vi "ImageManipulationNewLifetimeCalculation.vi"(0 "Array":T1[](array[typedef]) {"F2-Value overall" format="%.2f"; "tauerror" format="%.2f"; "Lifetime[ns]" format="%.2f"; "F2-Value TAC" format="%.2f"}, 1 "Decays":refnum<vi>, 2 "reference":refnum<vi>) -> ()   [LabVIEW 2009]
uses:
  spotproperties.ctl
panel:
  in  "OK Button":bool
  out "TAC intensity old":u32[](array[numeric])
  out "tauerror old":dbl[](array[numeric]) format="%.2f"
  out "Lifetime[ns] old":ext[](array[numeric]) format="%.2f"
  out "TAC intensity":u32[](array[numeric])
  out "tauerror":dbl[](array[numeric]) format="%.2f"
  out "Lifetime[ns]":ext[](array[numeric]) format="%.2f"
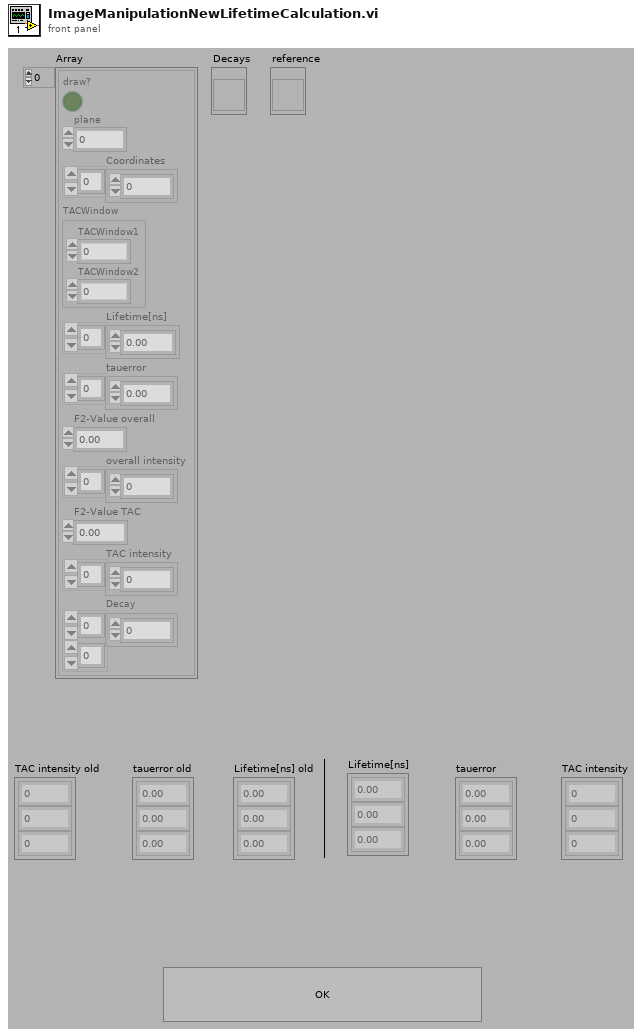
[diagram p1: front panel]
types:
  T1 = typedef "spotproperties.ctl" = cluster{"draw?":bool, "plane":u32, "Coordinates":i32[], "TACWindow":cluster{"TACWindow1":i32, "TACWindow2":i32}, "Lifetime[ns]":ext[], "tauerror":dbl[], "F2-Value overall":dbl, "overall intensity":u32[], "F2-Value TAC":dbl, "TAC intensity":u32[], "Decay":u32[][]}
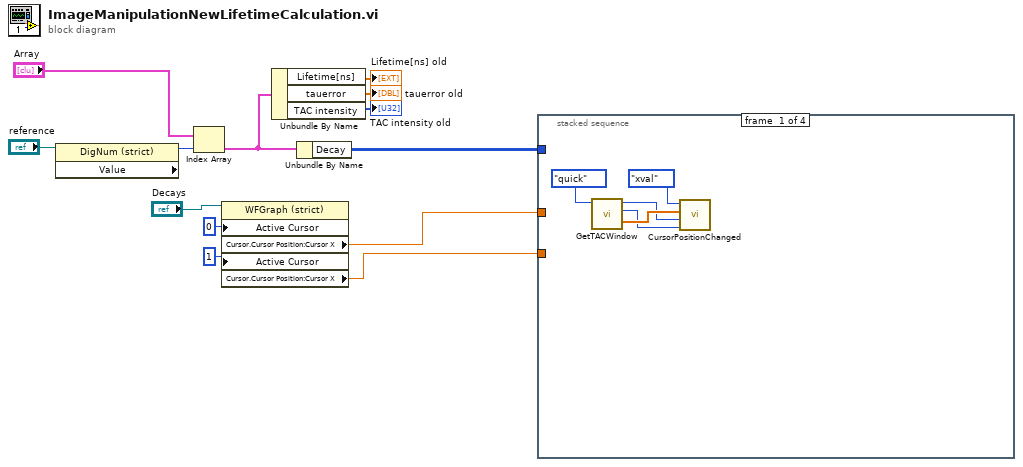
[diagram p0: block diagram]
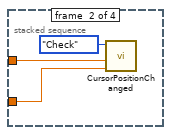
[diagram p2: hidden frame]
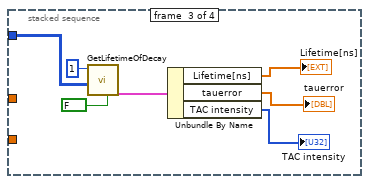
[diagram p3: hidden frame]
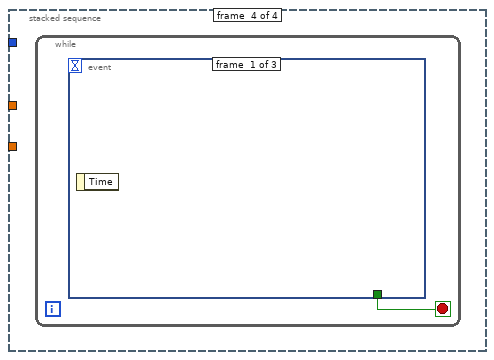
[diagram p4: hidden frame]
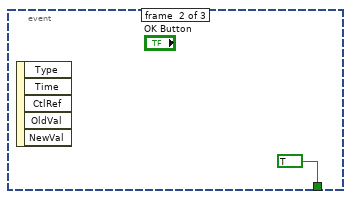
[diagram p5: hidden frame]
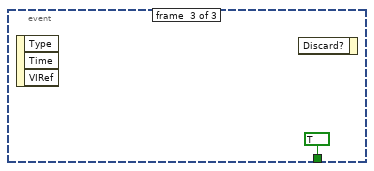
[diagram p6: hidden frame]
diagram:
  n1 = property on="Property Node" class="DigNum (strict)"(reference="reference") -> ("Value"=w7:u16)  [unwired: 1 in, 2 out]
  n2 = Index Array(array="Array", index=w7) -> (element=w4:T1)
  n3 = property class="WFGraph (strict)"(reference="Decays", "Active Cursor"=u32 0, "Active Cursor"=u32 1) -> ("Cursor.Cursor Position:Cursor X"=w12:dbl, "Cursor.Cursor Position:Cursor X"=w13:dbl)  [unwired: 1 in, 2 out]
  n4 = Unbundle By Name(w4) -> ("Lifetime[ns]"=→"Lifetime[ns] old":ext[], "tauerror"=→"tauerror old":dbl[], "TAC intensity"=→"TAC intensity old":u32[])
  n5 = Unbundle By Name(w4) -> ("Decay"=w11:u32[][])
  n6 = stacked-sequence {
    tunnel: w11 -> [_ _ w28 _]
    tunnel: w12 -> [_ w20 _ _]
    tunnel: w13 -> [_ w19 _ _]
    frame #0 {
      n7 = call "GetTACWindow.vi"("Enum"=enum16{"ini", "get", "quick"}."quick") -> ("Cursor.Cursor Position:Cursor X"=w15:u16, "Cursor.Cursor Position:Cursor X 2"=w14:u16, "x-values"=w17:dbl[])  [unwired: 1 in, 6 out]
      n8 = call "CursorPositionChanged.vi"("CursorPos x1"=w14, "CursorPos x0"=w15, "x-values"=w17, "action"=enum16{"Check", "Get", "xval"}."xval" ("Enum")) -> ()  [unwired: 4 out]
    }
    frame #1 {
      n9 = call "CursorPositionChanged.vi"("CursorPos x1"=w19, "CursorPos x0"=w20, "action"=enum16{"Check", "Get", "xval"}."Check" ("Enum")) -> ()  [unwired: 1 in, 4 out]
    }
    frame #2 {
      n10 = call "GetLifetimeOfDecay.vi"("F2-channel"=u8 1, "decay"=w28, "tauimage"=FALSE) -> ("SpotProperties"=w25:T1)  [unwired: 6 in]
      n11 = Unbundle By Name(w25) -> ("Lifetime[ns]"=→"Lifetime[ns]":ext[], "tauerror"=→"tauerror":dbl[], "TAC intensity"=→"TAC intensity":u32[])
    }
    frame #3 {
      n12 = while {
        stop <- w29 stop-if-true
        n13 = event shown="[2] Panel Close?" {
          selector: _ -> [_ _ _]
          dyn-events: _ -> [_ _ _]
          timeout: _ -> [_ _ _]
          tunnel: [_ TRUE TRUE] -> w29
          event #0 {
            n14 = event-data() -> ()  [unwired: 1 in, 1 out]
          }
          event #1 {
            n15 = event-data() -> ()  [unwired: 1 in, 5 out]
          }
          event #2 {
            n16 = event-data() -> ()  [unwired: 1 in, 3 out]
            n17 = event-data() -> ()  [unwired: 2 in, 1 out]
          }
        }
      }
    }
  }
